vi "Read Coils.vi"(8 "error in (no error)":errorcluster, 9 "number of coils":u16, 10 "starting address":u16, 11 "Modbus master in":refnum<class "Network Master.lvclass">) -> (0 "error out":errorcluster, 2 "coil values":bool[](array[boolean]), 3 "Modbus master out":refnum<class "Network Master.lvclass">)   [LabVIEW 2021, in "Network Master.lvclass"]
doc: "Reads values from contiguous coils. The maximum number of coils this VI can read is 2,000."
uses:
  Network Master.lvclass
  Modbus Data Unit/Modbus Data Unit.lvclass/Modbus Data Unit.ctl
  Network Master.lvclass/Network Master.ctl
  Modbus Data Unit/Construct PDU.vi
  Utility/Bytes to Bits.vi
  Data Model/Error Generator.vi
  Master Function Definition/Function code mismatch error.vi
  Modbus Data Unit/Deconstruct PDU.vi
  Modbus Data Unit/Modbus Data Unit.lvclass
  Transmission Data Unit/Transmission Data Unit.lvclass
  Master Function Definition/Master Function Definition.lvclass
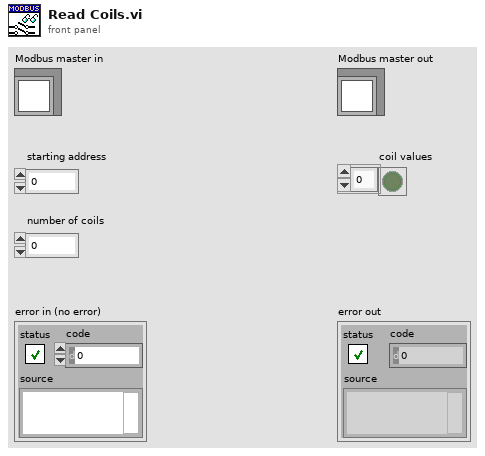
[diagram p1: front panel]
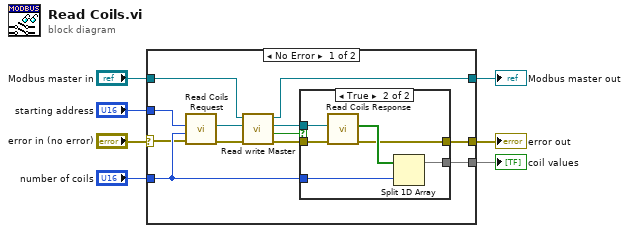
[diagram p0: block diagram]
diagram:
  n1 = case shown="No Error" "error in (no error)" {
    selector: "error in (no error)" -> [w8 w28]
    tunnel: [w15 w28] -> w5
    tunnel: [w9 w27] -> w6
    tunnel: "Modbus master in" -> [w10 w27]
    tunnel: "starting address" -> [w19 _]
    tunnel: "number of coils" -> [w18 _]
    tunnel: [w17 _] -> w4
    frame No Error {
      n2 = call "Read Coils Request.vi"("error in"=w8, "Number of coils"=w18, "Starting Address"=w19) -> ("error out"=w14:errorcluster, "modbus data unit out"=w11:refnum<class "Modbus Data Unit.lvclass">)  [unwired: 7 in]
      n3 = call "Read write Master.vi"("error in (no error)"=w14, "Modbus data unit in"=w11, "Modbus master in"=w10) -> ("error out"=w16:errorcluster, "PDU valid?"=w13:bool, "Modbus data unit out"=w12:refnum<class "Modbus Data Unit.lvclass">, "Modbus master out"=w9:refnum<class "Network Master.lvclass">)  [unwired: 5 in]
      n4 = case shown="True" w13 {
        tunnel: w18 -> [_ w26]
        tunnel: [_ w25] -> w17
        tunnel: w12 -> [_ w23]
        tunnel: w16 -> [w20 w22]
        tunnel: [w20 w21] -> w15
        frame False {
        }
        frame True {
          n5 = call "Read Coils Response.vi"("error in"=w22, "modbus data unit in"=w23) -> ("error out"=w21:errorcluster, "Data"=w24:bool[])  [unwired: 8 in]
          n6 = Split 1D Array(array=w24, index=w26) -> (first subarray=w25:bool[])  [unwired: 1 out]
        }
      }
    }
    frame Error {
    }
  }
  "error out" <- w5
  "Modbus master out" <- w6
  "coil values" <- w4
